vi "Read Measurement Osciloscope.vi"(8 "error in (no error)":errorcluster, 10 "Read Measurement In":T1={"TEKTRONIX- READ-IN"={"Channel (1: Channel 1)"=1, "Measurement Type (0: Frequency)"=0}, "EDU-X-1200A- READ-IN"={"Slope Type (0: Positive)"=0, "Measurement Type (0: Peak-Peak)"=0, "Occurrence Value (1)"=1, "Vertical Cross Value (0)"=0.0}} {"EDU-X-1200A- READ-IN"."Measurement Type (0: Peak-Peak)" items=["Peak-Peak", "Maximum", "Minimum", "Amplitude", "Top", "Base", "Overshoot", "Preshoot", "Average - N Cycles", "Average - Full Screen", "DC RMS - N Cycles", "DC RMS - Full Screen", "AC RMS - N Cycles", "AC RMS - Full Screen (Std Dev)", "Ratio", "Period", "Frequency", "Counter", "+Width", "-Width", "Burst Width", "Duty Cycle", "Rise Time", "Fall Time", "Delay", "Phase", "X minY", "X maxY", "Positive Pulse Count", "Negative Pulse Count", "Raising Edge Count", "Falling Edge Count", "Area - N Cycle", "Area - Full Screen", "Nth Edge Time", "Nth Edge Cross Level Time"]; "EDU-X-1200A- READ-IN"."Slope Type (0: Positive)" items=["Positive", "Negative"]; "TEKTRONIX- READ-IN"."Measurement Type (0: Frequency)" items=["Frequency", "Mean", "Period", "Pulse Duty", "Peak to Peak", "Cycle RMS", "Minimum", "Maximum", "Rise Time", "Fall Time", "Positive Width", "Negative Width", "Amplitude", "Cycle Mean", "High", "Low", "Negative Duty", "Positive Overshoot", "Negative Overshoot", "Cursor Mean", "Burst Width", "Positive Pulse Count", "Negative Pulse Count", "Rising Edge Count", "Falling Edge Count", "Area", "Cycle Area", "RMS", "Cursor RMS"]; "TEKTRONIX- READ-IN"."Channel (1: Channel 1)" items=["Channel 1"=1, "Channel 2"=2, "Channel 3"=3, "Channel 4"=4]}, 11 "Tektronicks in":refnum<class "Tektronicks.lvclass">) -> (0 "error out":errorcluster, 2 "Read measurement Out":T2, 3 "Tektronicks out":refnum<class "Tektronicks.lvclass">)   [LabVIEW 2020, in "Tektronicks.lvclass"]
uses:
  Tektronicks.lvclass
  TypeDefs/ReadMeasurementOut--cluster.ctl
  TypeDefs/ReadMeasurementIn--cluster.ctl
  Tektronicks.lvclass/Tektronicks.ctl
  <instrlib>/Tektronix TDS 200 1000 2000 Series/Tektronix TDS 200 1000 2000 Series.lvlib
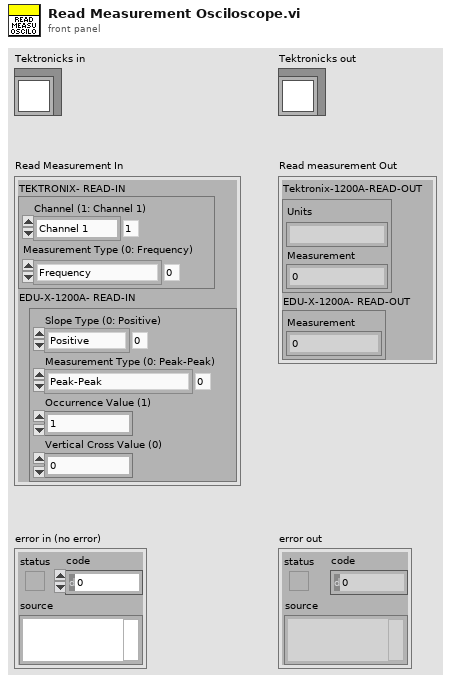
[diagram p1: front panel]
types:
  T1 = typedef "ReadMeasurementIn--cluster.ctl" = cluster{"TEKTRONIX- READ-IN":cluster{"Channel (1: Channel 1)":i32, "Measurement Type (0: Frequency)":i32}, "EDU-X-1200A- READ-IN":cluster{"Slope Type (0: Positive)":i32, "Measurement Type (0: Peak-Peak)":i32, "Occurrence Value (1)":i32, "Vertical Cross Value (0)":dbl}}
  T2 = typedef "ReadMeasurementOut--cluster.ctl" = cluster{"Tektronix-1200A-READ-OUT":cluster{"Units":string, "Measurement":dbl}, "EDU-X-1200A- READ-OUT":cluster{"Measurement":dbl}}
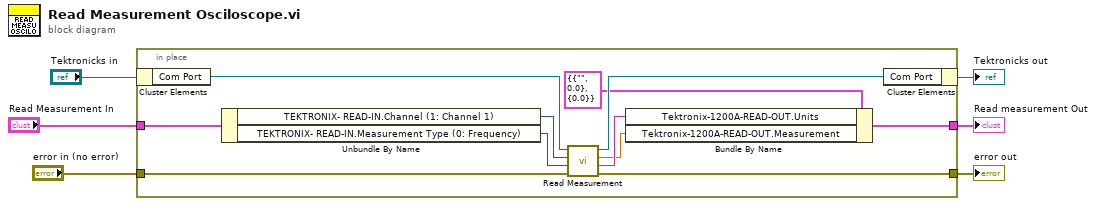
[diagram p0: block diagram]
diagram:
  n1 = in-place {
    in-place-border: "error in (no error)" -> [w15]
    in-place-border: [w14] -> w3
    in-place-border: "Read Measurement In" -> [w13]
    in-place-border: [w9] -> w1
    n2 = in-place-cluster #1("Tektronicks in") -> ("Com Port"=w17:refnum<visa-resource-name>)
    n3 = Unbundle By Name(w13) -> ("TEKTRONIX- READ-IN.Channel (1: Channel 1)"=w12:i32, "TEKTRONIX- READ-IN.Measurement Type (0: Frequency)"=w11:i32)
    n4 = call <instrlib>:"Read Measurement.vi"("error in (no error)"=w15, "Measurement Type (0: Frequency)"=w11, "Channel (1: Channel 1)"=w12, "VISA resource name"=w17) -> ("error out"=w14:errorcluster, "Units"=w8:string, "Measurement"=w7:dbl, "VISA resource name out"=w16:refnum<visa-resource-name>)  [unwired: 4 in]
    n5 = Bundle By Name(cluster=T2 {"Tektronix-1200A-READ-OUT"={"Units"="", "Measurement"=0.0}, "EDU-X-1200A- READ-OUT"={"Measurement"=0.0}} ("Read measurement Out"), "Tektronix-1200A-READ-OUT.Units"=w8, "Tektronix-1200A-READ-OUT.Measurement"=w7) -> (w9:T2)
    n6 = in-place-cluster #1("Com Port"=w16) -> (→"Tektronicks out":refnum<class "Tektronicks.lvclass">)
  }
  "error out" <- w3
  "Read measurement Out" <- w1
